vi "get_plot_y_scale_data.vi"(10 "plot_selector":string, 11 "cursor_value_in":dbl) -> (2 "prefix/unit":string, 3 "cursor_value_out":dbl)   [LabVIEW 2025]
uses:
  00_global_variables.vi
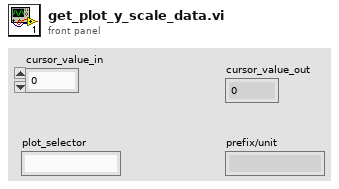
[diagram p1: front panel]
types:
  T1 = cluster{"y_scale_id":u32, "unit":string, "prefix_enable":bool, "plot_id":u32}[]
  T2 = cluster{"y_scale_id":u32, "unit":string, "prefix_enable":bool, "plot_id":u32}
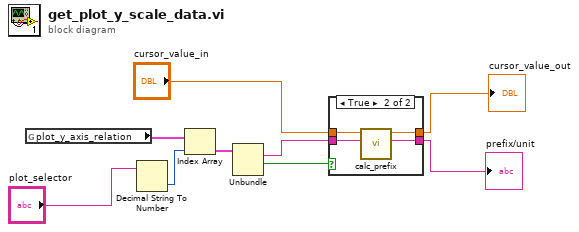
[diagram p0: block diagram]
diagram:
  n1 = global read "00_global_variables.vi" "plot_y_axis_relation"() -> (w2:T1)
  n2 = Decimal String To Number(string="plot_selector") -> (number=w7:i32)  [unwired: 2 in, 1 out]
  n3 = Index Array(array=w2, index=w7) -> (element=w9:T2)
  n4 = Unbundle(w9) -> ("unit"=w8:string, "prefix_enable"=w6:bool)  [unwired: 2 out]
  n5 = case shown="True" w6 {
    tunnel: [w11 w15] -> w4
    tunnel: [w10 w14] -> w5
    tunnel: w8 -> [w10 w13]
    tunnel: "cursor_value_in" -> [w11 w12]
    frame False {
    }
    frame True {
      n6 = call "calc_prefix.vi"("unit"=w13, "Numeric in"=w12) -> ("prefix"=w14:string, "Numeric out"=w15:dbl)  [unwired: 8 in]
    }
  }
  "prefix/unit" <- w5
  "cursor_value_out" <- w4
